vi "LVTest.vi"() -> ()   [LabVIEW 2017]
uses:
  cmake-build-release/Database.dll
panel:
  out "arg1":string[](array[string])
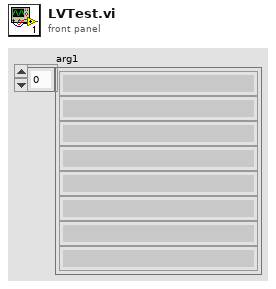
[diagram p1: front panel]
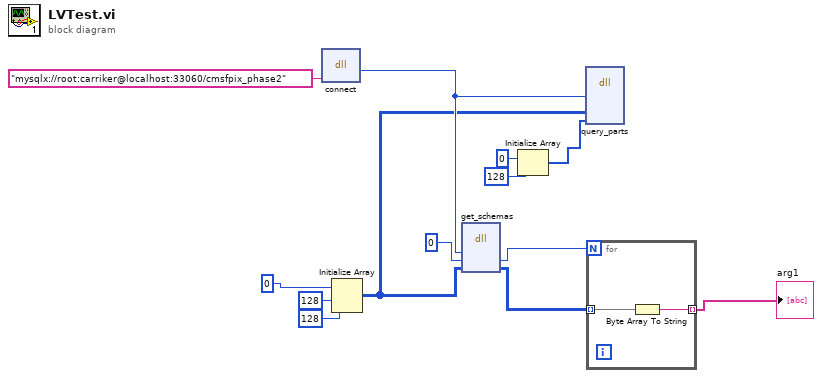
[diagram p0: block diagram]
diagram:
  n1 = dll-call lib="C:/Users/Caleb/Desktop/CLionLVTest/cmake-build-release/Database.dll" fn="connect"("conn_str"="mysqlx://root:carriker@localhost:33060/cmsfpix_phase2") -> ("return type"=w5:i32)  [unwired: 4 in, 2 out]
  n2 = Initialize Array(u8 0, 128 ("dimension size"), 128 ("dimension size")) -> (w4:u8[][])
  n3 = dll-call lib="C:/Users/Caleb/Desktop/CLionLVTest/cmake-build-release/Database.dll" fn="get_schemas"("session_id"=w5, "n_schemas"=0, "schemas"=w4) -> ("n_schemas"=w7:i32, "schemas"=w8:u8[][])  [unwired: 5 in, 2 out]
  n4 = Initialize Array(0 ("element"), 128 ("dimension size")) -> (w1:i32[])
  n5 = dll-call lib="C:/Users/Caleb/Desktop/CLionLVTest/cmake-build-release/Database.dll" fn="query_parts"("session_id"=w5, "part"=w4, "version"=w1) -> ()  [unwired: 9 in, 2 out]
  n6 = for {
    N: w7 -> [_]
    tunnel: w8 -> [w15] mode=indexing
    tunnel: [w14] -> w6 mode=indexing
    n7 = Byte Array To String(unsigned byte array=w15) -> (string=w14:string)
  }
  "arg1" <- w6
